vi "array_light_mix_tap_duration_details.vi"() -> ()   [LabVIEW 2014]
panel:
  in  "Light stim duration (Frames)":dbl[](array[numeric])
  in  "Power Array (uW/mm^2)":dbl[](array[numeric])
  in  "Proportion of cycles with no tap":dbl
  in  "Proportion of cycles with no light":dbl
  in  "Light ON duration after tap (frames)":dbl
  in  "Period per cycle (frames)":dbl
  in  "Taps per cycle (count)":i32
  in  "Total duration (frames)":dbl
  out "Frames":i32
  in  "Transfer and Run Date Folder After Experiment":bool
  in  "SSH user name":string
  in  "SSH password":string
  in  "Wait before recording (s)":dbl
  in  "Tags":string
  in  "Start Recording":bool
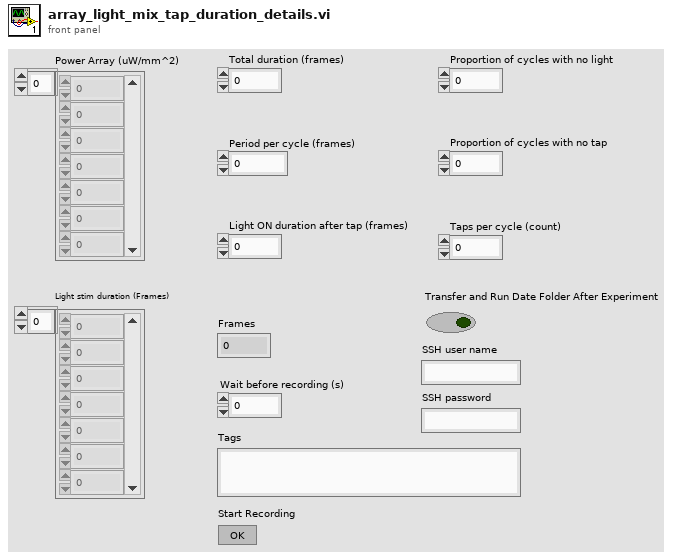
[diagram p1: front panel]
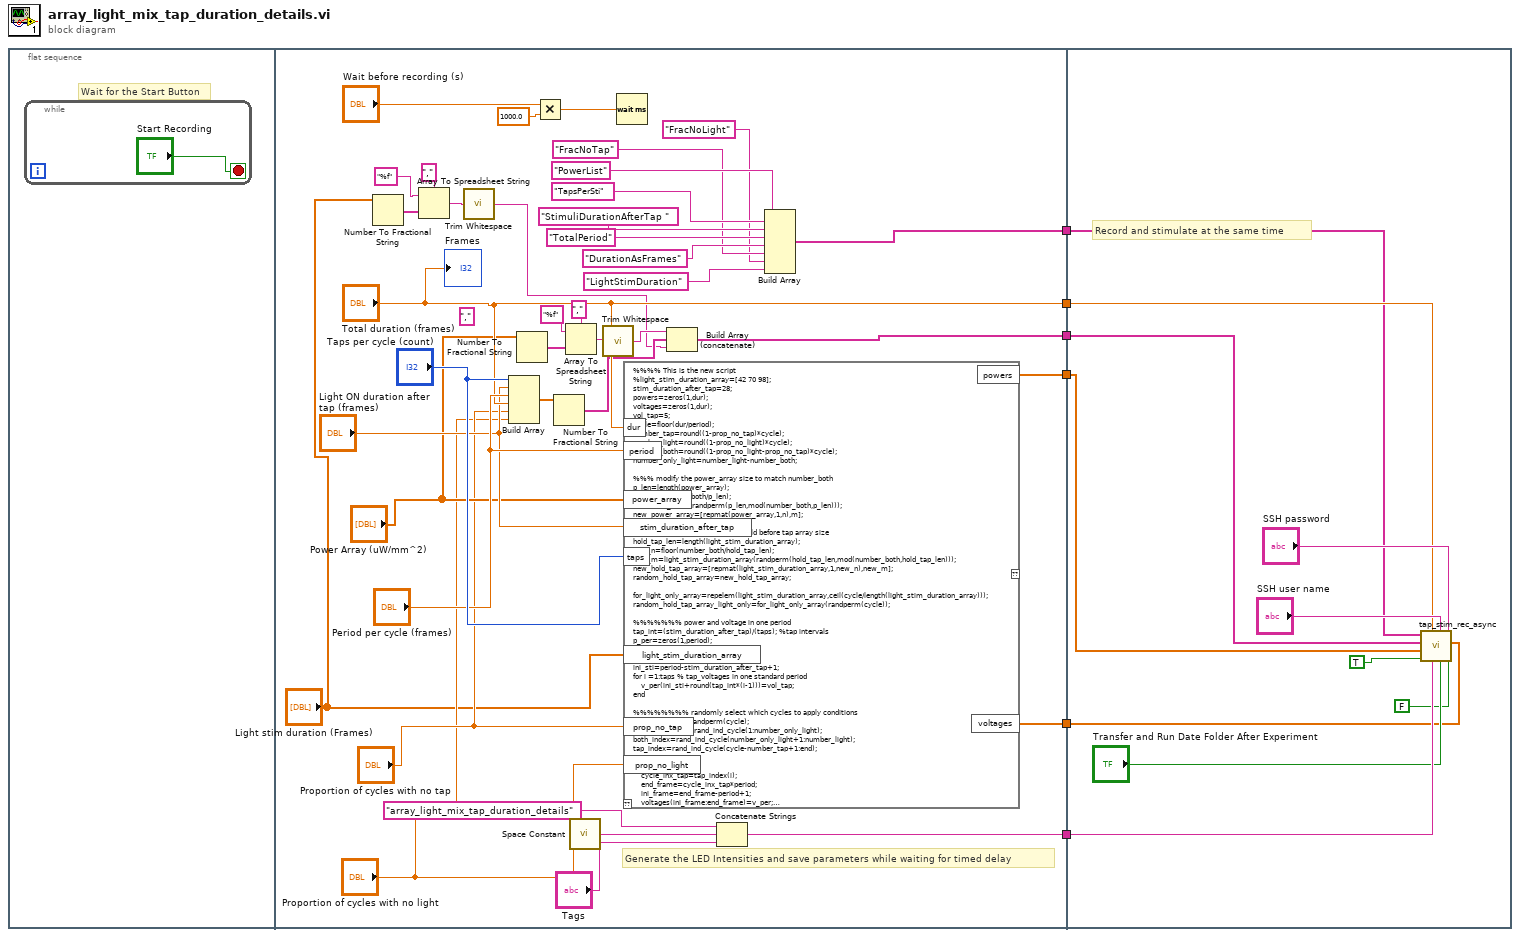
[diagram p0: block diagram]
diagram:
  n1 = flat-sequence {
    tunnel: [w43] -> w6
    tunnel: [w37] -> w5
    tunnel: ["Total duration (frames)"] -> w4
    tunnel: [w15] -> w3
    tunnel: [w33] -> w2
    tunnel: [w25] -> w1
    tunnel: w6 -> [w57]
    tunnel: w5 -> [w49]
    tunnel: w4 -> [w53]
    tunnel: w3 -> [w52]
    tunnel: w2 -> [w48]
    tunnel: w1 -> [w47]
    frame #0 {
      # "Wait for the Start Button"
      n2 = while {
        stop <- "Start Recording" stop-if-true
      }
    }
    frame #1 {
      (unwired) ","
      # "Generate the LED Intensities and save parameters while waiting for timed delay"
      n3 = Number To Fractional String(number="Light stim duration (Frames)") -> (F-format string=w12:string[])  [unwired: 3 in]
      n4 = Array To Spreadsheet String(delimiter (Tab)=",", array=w12, 3:"%f") -> (spreadsheet string=w9:string)
      n5 = call <vilib>:"Trim Whitespace.vi"("string"=w9) -> ("trimmed string"=w8:string)  [unwired: 1 in]
      n6 = Build Array("Taps per cycle (count)", "Light ON duration after tap (frames)", "Period per cycle (frames)", "Total duration (frames)", "Proportion of cycles with no tap", "Proportion of cycles with no light") -> (w36:dbl[])
      n7 = Number To Fractional String(number="Power Array (uW/mm^2)") -> (F-format string=w20:string[])  [unwired: 3 in]
      n8 = Multiply(x="Wait before recording (s)", y=1000.0) -> (x*y=w41:dbl)
      n9 = Number To Fractional String(number=w36) -> (F-format string=w26:string[])  [unwired: 3 in]
      n10 = Array To Spreadsheet String(delimiter (Tab)=",", array=w20, 3:"%f") -> (spreadsheet string=w30:string)
      n11 = call <vilib>:"Space Constant.vi"() -> ("String"=w45:string)
      n12 = call <vilib>:"Trim Whitespace.vi"("string"=w30) -> ("trimmed string"=w27:string)  [unwired: 1 in]
      n13 = Wait (ms)(milliseconds to wait=w41) -> ()  [unwired: 1 out]
      n14 = script code="%%%% This is the new script\n%light_stim_duration_array=[42 70 98];\nstim_duration_after_tap=28;\npowers=zeros(1,dur);\nvoltages=zeros(1,dur);\nvol_tap=5;\ncycle=floor(dur/period);\nnumber_tap=round((1-prop_no_tap)*cycle);\nnumber_light=round((1-prop_no_light)*cycle);\nnumber_both=round((1-prop_no_light-prop_no_tap)*cycle);\nnumber_only_light=number_light-number_both;\n\n%%% modify the power_array size to match number_both\np_len=length(power_array);\nn=floor(number_both/p_len);\nm=power_array(randperm(p_len,mod(number_both,p_len)));\nnew_power_array=[repmat(power_array,1,n),m];\n\n%%%%%%%%%% modify the hold before tap array size \nhold_tap_len=length(light_stim_duration_array);\nnew_n=floor(number_both/hold_tap_len);\nnew_m=light_stim_duration_array(randperm(hold_tap_len,mod(number_both,hold_tap_len)));\nnew_hold_tap_array=[repmat(light_stim_duration_array,1,new_n),new_m];\nrandom_hold_tap_array=new_hold_tap_array;\n\nfor_light_only_array=repelem(light_stim_duration_array,ceil(cycle/length(light_stim_duration_array)));\nrandom_hold_tap_array_light_only=for_light_only_array(randperm(cycle));\n\n%%%%%%% power and voltage in one period\ntap_int=(stim_duration_after_tap)/(taps); %tap intervals\np_per=zeros(1,period);\nv_per=zeros(1,period);\n\nini_sti=period-stim_duration_after_tap+1;\nfor i =1:taps % tap_voltages in one standard period\n    v_per(ini_sti+round(tap_int*(i-1)))=vol_tap;\nend\n\n%%%%%%%% randomly select which cycles to apply conditions\nrand_ind_cycle=randperm(cycle);\nlight_only_index=rand_ind_cycle(1:number_only_light);\nboth_index=rand_ind_cycle(number_only_light+1:number_light);\ntap_index=rand_ind_cycle(cycle-number_tap+1:end);\n\nfor i=1:number_tap\n    cycle_inx_tap=tap_index(i);\n    end_frame=cycle_inx_tap*period;\n    ini_frame=end_frame-period+1;\n    voltages(ini_frame:end_frame)=v_per;\nend\n\nfor i=1:number_both\n    \n    cycle_inx_both=tap_index(i);\n    end_frame=cycle_inx_both*period;\n    ini_frame=end_frame-period+1;\n    voltages(ini_frame:end_frame)=v_per;\n        \n    ini_sti=period-random_hold_tap_array(i)+1;\n    p_per(ini_sti:period)=1;\n        \n    cycle_inx_both=both_index(i);\n    power=new_power_array(i);\n    end_frame=cycle_inx_both*period;\n    ini_frame=end_frame-period+1;\n    powers(ini_frame:end_frame)=p_per.*power;\n    p_per=zeros(1,period);\nend\n\n%%%%%% for_light_only=[repmat(power_array,1, round(cycle/p_len)),[]];\nfor_light_only=repelem(power_array,ceil(cycle/p_len));\npower_array_light_only=for_light_only(randperm(cycle));\n\nfor i=1:number_only_light\n    cycle_inx_light=light_only_index(i);\n    power=power_array_light_only(i);\n    end_frame=cycle_inx_light*period;\n    ini_frame=end_frame-period+1;\n    \n    ini_sti=period-random_hold_tap_array_light_only(i)+1;\n    p_per(ini_sti:period)=1;\n    powers(ini_frame:end_frame)=p_per.*power;\n    p_per=zeros(1,period);\nend"("taps"="Taps per cycle (count)", "stim_duration_after_tap"="Light ON duration after tap (frames)", "period"="Period per cycle (frames)", "dur"="Total duration (frames)", "prop_no_tap"="Proportion of cycles with no tap", "prop_no_light"="Proportion of cycles with no light", "power_array"="Power Array (uW/mm^2)", "light_stim_duration_array"="Light stim duration (Frames)") -> ("powers"=w15:dbl[], "voltages"=w33:dbl[])  [unwired: 1 in, 1 out]
      n15 = Build Array (concatenate)(w27, w26, w8) -> (w25:string[])
      n16 = Concatenate Strings("array_light_mix_tap_duration_details", w45, "Tags") -> (w43:string)
      n17 = Build Array("PowerList", "TapsPerSti", "StimuliDurationAfterTap ", "TotalPeriod", "DurationAsFrames", "FracNoTap", "FracNoLight", "LightStimDuration") -> (w37:string[])
      "Frames" <- "Total duration (frames)"
    }
    frame #2 {
      # "Record and stimulate at the same time"
      n18 = call "tap_stim_rec_async.vi"("Convert Power to Voltage B"=FALSE, "voltages/power B"=w48, "SSH password"="SSH password", "Transfer and Run Date Folder After Experiment"="Transfer and Run Date Folder After Experiment", "SSH user name"="SSH user name", "Tags"=w57, "Frames"=w53, "Convert Power to Voltage"=TRUE, "voltages/power A"=w52, "parameters"=w47, "parameters headers"=w49) -> ()  [unwired: 1 in]
    }
  }
